vi "Make DLL Param Advanced(Profile Rsp).vi"   [LabVIEW 8.6, in "Keyence LJ-V7000.lvlib"]
uses:
  Keyence LJ-V7000.lvlib
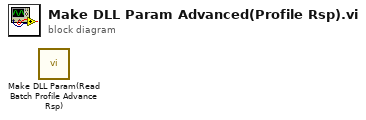
[diagram p0: block diagram]
diagram:
  n1 = call "Make DLL Param(Read Batch Profile Advance Rsp).vi"() -> ()  [unwired: 1 in, 1 out]
